vi "test child test method.vi"(8 "error in (no error)":errorcluster, 11 "VI tester Child in":refnum<class "VI tester Child.lvclass">) -> (0 "error out":errorcluster, 3 "VI tester Child out":refnum<class "VI tester Child.lvclass">)   [LabVIEW 2020, in "VI tester Child.lvclass"]
uses:
  VI tester Child.lvclass
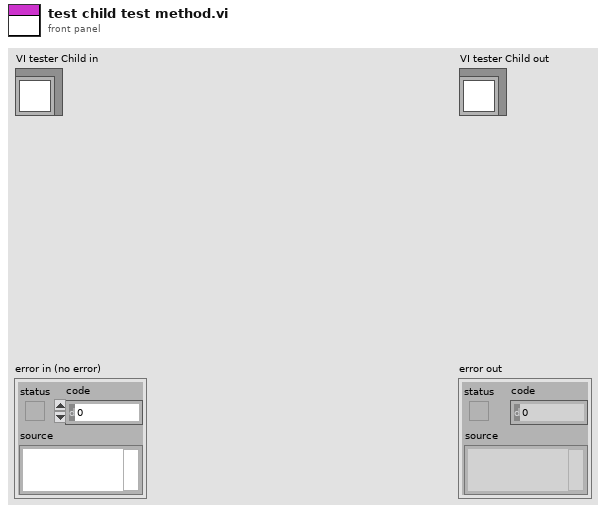
[diagram p1: front panel]
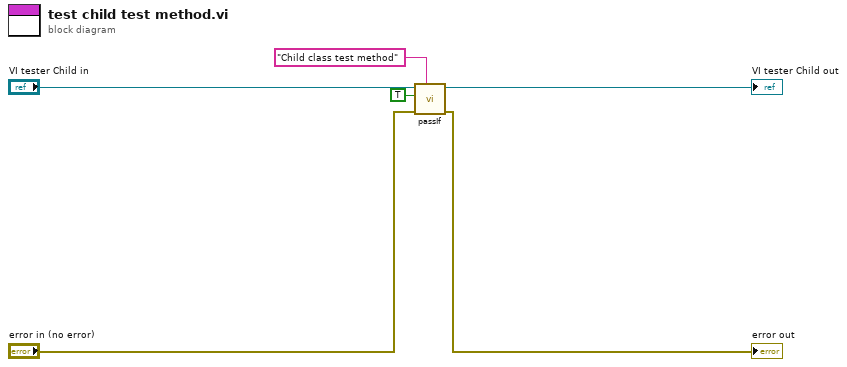
[diagram p0: block diagram]
diagram:
  n1 = call-dynamic "passIf.vi"("custom report message (\"\")"="Child class test method" ("custom report message (\"\")"), "error in (no error)"="error in (no error)", "pass"=TRUE, "TestCase in"="VI tester Child in") -> ("error out"=→"error out":errorcluster, "TestCase out"=→"VI tester Child out":refnum<class "VI tester Child.lvclass">)  [unwired: 6 in]
